vi "CLI Build from Project Path.vi"() -> ()   [LabVIEW 2020, in "ProjectBuilder.lvlib"]
uses:
  ProjectBuilder.lvlib
  PPL/HDH.ClassLoader.lvlibp
panel:
  out "Quit after execution?":bool
  out "Valid project?":bool
  out "Project path":path
  # "Running 'Build Project' on:"
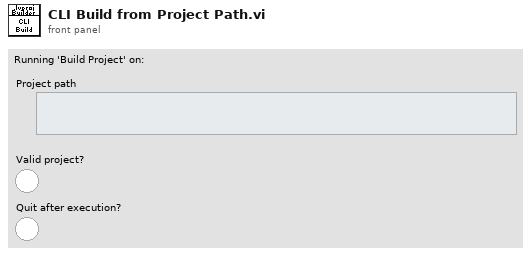
[diagram p1: front panel]
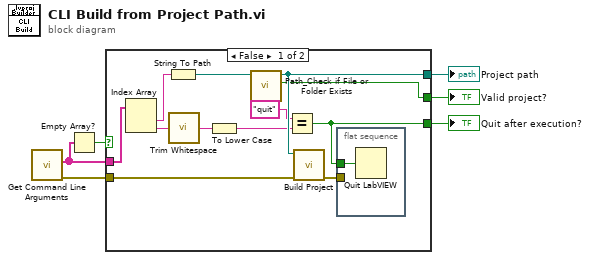
[diagram p0: block diagram]
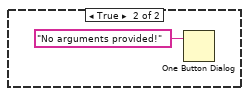
[diagram p2: hidden frame]
diagram:
  n1 = call <vilib>:"Get Command Line Arguments.vi"() -> ("error out"=w6:errorcluster, "arguments"=w2:string[])  [unwired: 9 in, 1 out]
  n2 = Empty Array?(array=w2) -> (empty?=w1:bool)
  n3 = case shown="False" w1 {
    tunnel: w6 -> [w18 _]
    tunnel: [w13 _] -> w5
    tunnel: [w12 _] -> w4
    tunnel: [w8 _] -> w3
    tunnel: w2 -> [w7 _]
    frame False {
      n4 = Index Array(array=w7) -> (element #1=w17:string, element #2=w15:string)  [unwired: 2 in]
      n5 = String To Path(string=w17) -> (path=w14:path)
      n6 = call <vilib>:"Trim Whitespace.vi"("string"=w15) -> ("trimmed string"=w11:string)  [unwired: 1 in]
      n7 = To Lower Case(string=w11) -> (all lower case string=w10:string)
      n8 = call "Path_Check if File or Folder Exists.vi"("File or Folder Path in"=w14) -> ("File or Folder Found?"=w12:bool, "File or Folder Path dub"=w13:path)  [unwired: 9 in]
      n9 = Equal?(x="quit", y=w10) -> (x = y?=w8:bool)
      n10 = call "Build Project.vi"("error in (no error)"=w18, "Project Path"=w13) -> ("error out"=w16:errorcluster)  [unwired: 7 in, 2 out]
      n11 = flat-sequence {
        tunnel: w16 -> [_]
        tunnel: w8 -> [w19]
        frame #0 {
          n12 = Quit LabVIEW(quit? (T)=w19) -> ()
        }
      }
    }
    frame True {
      n13 = One Button Dialog(message="No arguments provided!") -> ()  [unwired: 1 in, 1 out]
    }
  }
  "Project path" <- w5
  "Valid project?" <- w4
  "Quit after execution?" <- w3
